vi "Number of Results.vi"() -> (2 "number of methods":i32=2, 3 "number of results":i32=2)   [LabVIEW 2020, in "Light Test Case Double Copy.lvclass"]
uses:
  Light Test Case Double Copy.lvclass
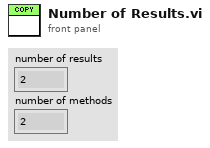
[diagram p1: front panel]
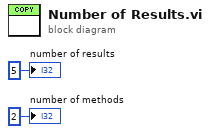
[diagram p0: block diagram]
diagram:
  "number of results" <- 5 ("y")
  "number of methods" <- 2 ("number of methods")
